vi "Optoelectronic Loop.vi"(8 "error in":errorcluster, 10 "Message Queues out":T14, 11 "Notifiers":T1) -> (0 "error out":errorcluster)   [LabVIEW 2014]
uses:
  support/Message Queue/All Message Queues.ctl
  support/Message Queue/Message Cluster.ctl
  support/Notifiers/Notifiers.ctl
  support/Message Handler Loop Notifiers.ctl
  Hardware Control/Parameter Analyzer/Parameter Analyzer Notifiers.ctl
  Hardware Control/Switching Matrix/Switching Matrix Notifiers.ctl
  Hardware Control/Stress Control/StressControl Notifiers.ctl
  Hardware Control/Spectrometer/Spectrometer Notifiers.ctl
  Hardware Control/Switches and Mirrors/SwitchesMirrors Notifiers.ctl
  Hardware Control/Camera/Camera Notifiers.ctl
  Hardware Control/XYZ Stage/XYZ Notifications.ctl
  Hardware Control/Autofocus/Autofocus Notifiers.ctl
  Measurements/Optoelectronic Measurement/Optoelectronic Notifiers.ctl
  Measurements/Save Data/SaveData Notifiers.ctl
  Measurements/Instrument Sequence/Instrument Sequence Notifiers.ctl
  Measurements/Optoelectronic Measurement/Optoelectronic Funtions.ctl
  support/Message Queue/Message Queue.lvlib
panel:
  # "LICENSED MATERIALS – PROPERTY OF IBM\nCopyright IBM Corp. 2016,\nALL RIGHTS RESERVED"
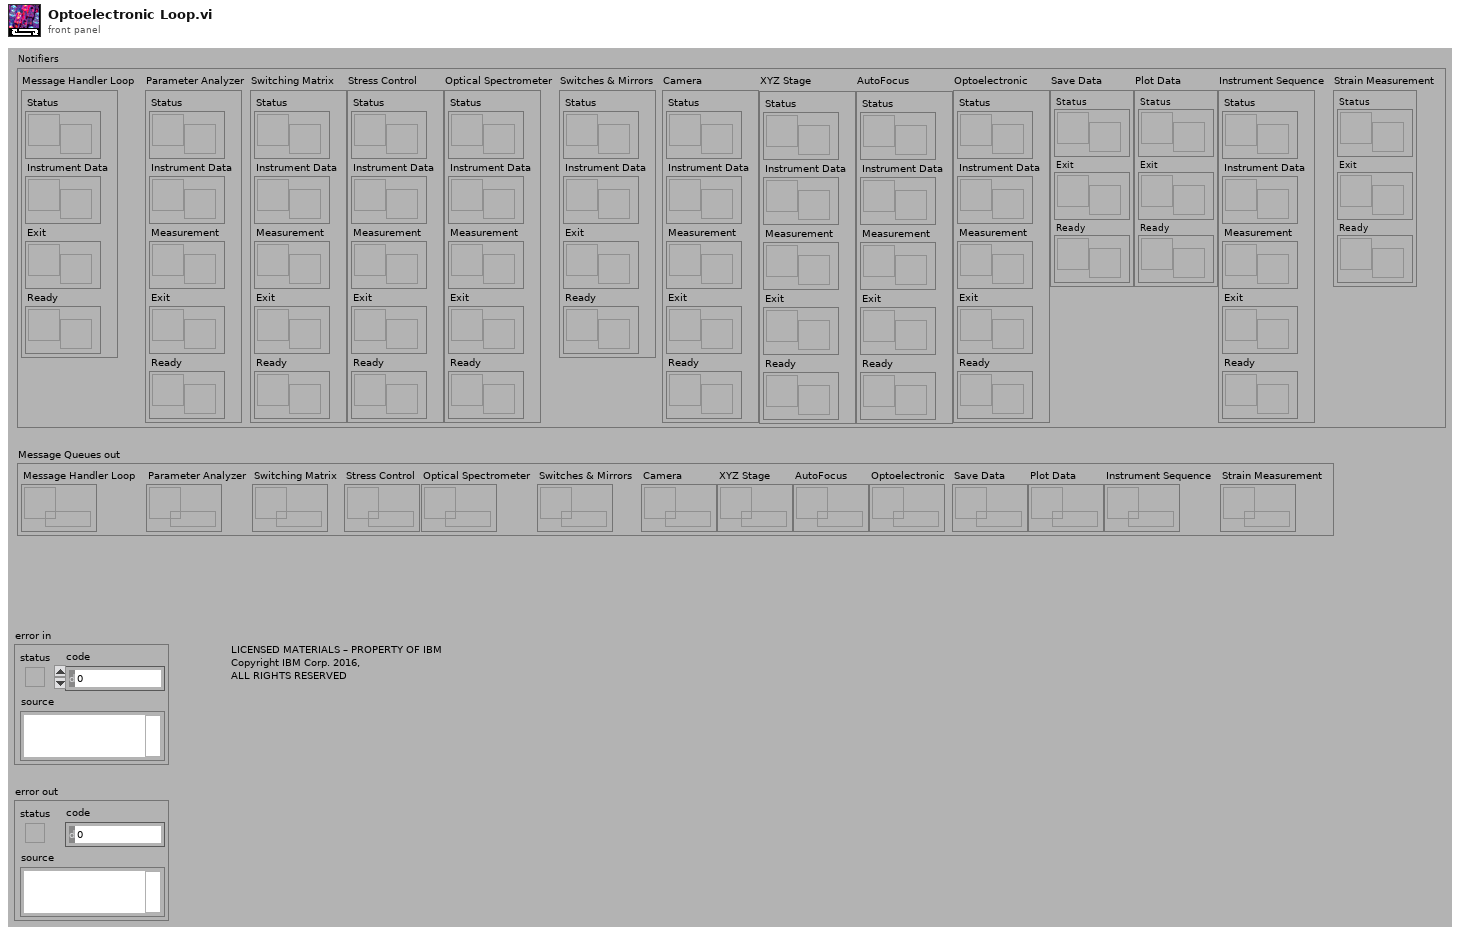
[diagram p1: front panel]
types:
  T1 = typedef "Notifiers.ctl" = cluster{"Message Handler Loop":T2, "Parameter Analyzer":T3, "Switching Matrix":T4, "Stress Control":T5, "Optical Spectrometer":T6, "Switches & Mirrors":T7, "Camera":T8, "XYZ Stage":T9, "AutoFocus":T10, "Optoelectronic":T11, "Save Data":T12, "Plot Data":T12, "Instrument Sequence":T13, "Strain Measurement":cluster{"Status":refnum<notifier>, "Exit":refnum<notifier>, "Ready":refnum<notifier>}}
  T2 = typedef "Message Handler Loop Notifiers.ctl" = cluster{"Status":refnum<notifier>, "Instrument Data":refnum<notifier>, "Exit":refnum<notifier>, "Ready":refnum<notifier>}
  T3 = typedef "Parameter Analyzer Notifiers.ctl" = cluster{"Status":refnum<notifier>, "Instrument Data":refnum<notifier>, "Measurement":refnum<notifier>, "Exit":refnum<notifier>, "Ready":refnum<notifier>}
  T4 = typedef "Switching Matrix Notifiers.ctl" = cluster{"Status":refnum<notifier>, "Instrument Data":refnum<notifier>, "Measurement":refnum<notifier>, "Exit":refnum<notifier>, "Ready":refnum<notifier>}
  T5 = typedef "StressControl Notifiers.ctl" = cluster{"Status":refnum<notifier>, "Instrument Data":refnum<notifier>, "Measurement":refnum<notifier>, "Exit":refnum<notifier>, "Ready":refnum<notifier>}
  T6 = typedef "Spectrometer Notifiers.ctl" = cluster{"Status":refnum<notifier>, "Instrument Data":refnum<notifier>, "Measurement":refnum<notifier>, "Exit":refnum<notifier>, "Ready":refnum<notifier>}
  T7 = typedef "SwitchesMirrors Notifiers.ctl" = cluster{"Status":refnum<notifier>, "Instrument Data":refnum<notifier>, "Exit":refnum<notifier>, "Ready":refnum<notifier>}
  T8 = typedef "Camera Notifiers.ctl" = cluster{"Status":refnum<notifier>, "Instrument Data":refnum<notifier>, "Measurement":refnum<notifier>, "Exit":refnum<notifier>, "Ready":refnum<notifier>}
  T9 = typedef "XYZ Notifications.ctl" = cluster{"Status":refnum<notifier>, "Instrument Data":refnum<notifier>, "Measurement":refnum<notifier>, "Exit":refnum<notifier>, "Ready":refnum<notifier>}
  T10 = typedef "Autofocus Notifiers.ctl" = cluster{"Status":refnum<notifier>, "Instrument Data":refnum<notifier>, "Measurement":refnum<notifier>, "Exit":refnum<notifier>, "Ready":refnum<notifier>}
  T11 = typedef "Optoelectronic Notifiers.ctl" = cluster{"Status":refnum<notifier>, "Instrument Data":refnum<notifier>, "Measurement":refnum<notifier>, "Exit":refnum<notifier>, "Ready":refnum<notifier>}
  T12 = typedef "SaveData Notifiers.ctl" = cluster{"Status":refnum<notifier>, "Exit":refnum<notifier>, "Ready":refnum<notifier>}
  T13 = typedef "Instrument Sequence Notifiers.ctl" = cluster{"Status":refnum<notifier>, "Instrument Data":refnum<notifier>, "Measurement":refnum<notifier>, "Exit":refnum<notifier>, "Ready":refnum<notifier>}
  T14 = typedef "Message Queue.lvlib/All Message Queues.ctl" = cluster{"Message Handler Loop":refnum<queue>, "Parameter Analyzer":refnum<queue>, "Switching Matrix":refnum<queue>, "Stress Control":refnum<queue>, "Optical Spectrometer":refnum<queue>, "Switches & Mirrors":refnum<queue>, "Camera":refnum<queue>, "XYZ Stage":refnum<queue>, "AutoFocus":refnum<queue>, "Optoelectronic":refnum<queue>, "Save Data":refnum<queue>, "Plot Data":refnum<queue>, "Instrument Sequence":refnum<queue>, "Strain Measurement":refnum<queue>}
  T15 = typedef "Optoelectronic Data.ctl" = cluster{"Refnums":T16, "Initialize":T19}
  T16 = typedef "Optoelectronic Refnums.ctl" = cluster{"Instrument Status":refnum<vi>, "Optical Spectrum Plot":T17, "Electrical Data Plot":T18}
  T17 = typedef "Optical Spectrum Plot Refnum.ctl" = cluster{"Plot List":refnum<vi>, "Optical Spectrum vs Energy":refnum<vi>, "Optical Spectrum vs Wavelength":refnum<vi>, "Optical Spectrum vs Raman Shift":refnum<vi>, "Detector Temperature":refnum<vi>}
  T18 = typedef "Electrical Data Plot Refnums.ctl" = cluster{"Plot List":refnum<vi>, "Voltage Plot":refnum<vi>, "Current Plot":refnum<vi>, "IV Characteristic":refnum<vi>, "dI/dV-V Characteristic":refnum<vi>}
  T19 = typedef "Optoelectronic Initialize.ctl" = cluster{"Update Refnums":bool}
  T20 = typedef "Optoelectronic Funtions.ctl" = enum16{"Get Instruments Status", "Measure", "Set Parameter Analyzer", "Set Spectrometer", "Set Acquisition", "Update Refnums"}
  T21 = typedef "SaveData Workspace Info.ctl" = cluster{"Device Name":string, "Device Info":string, "Path":path}
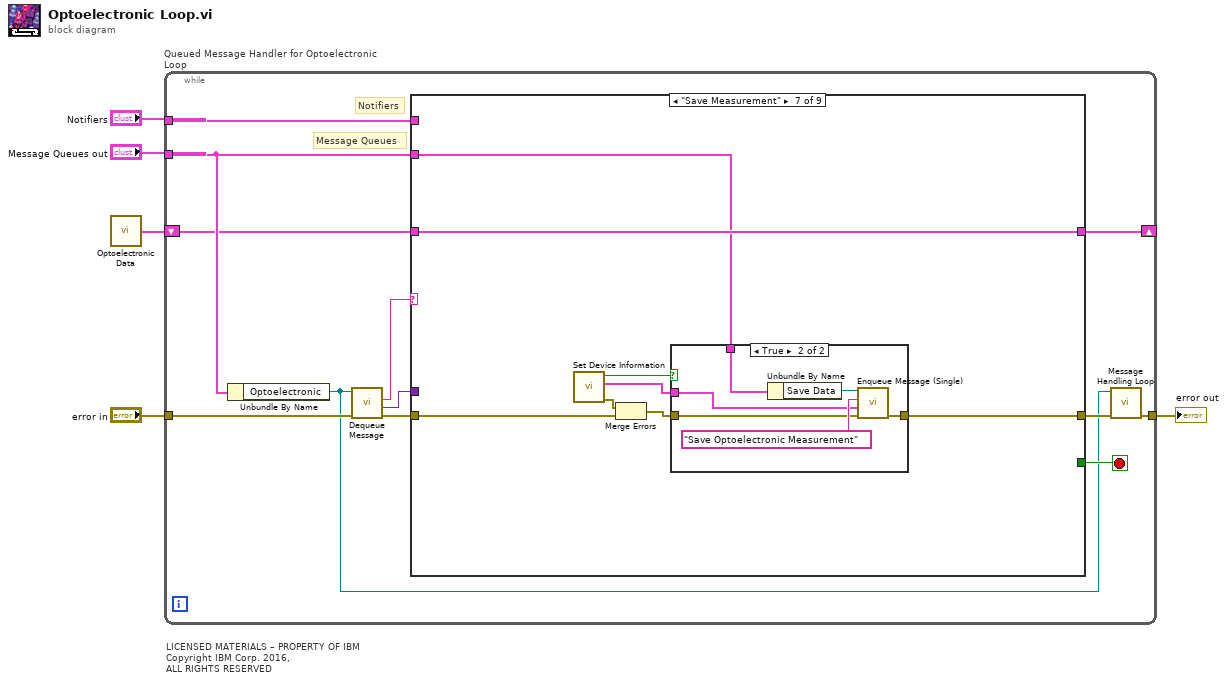
[diagram p0: block diagram]
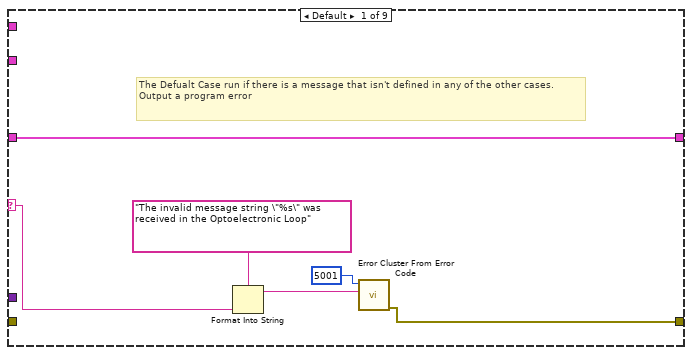
[diagram p2: hidden frame]
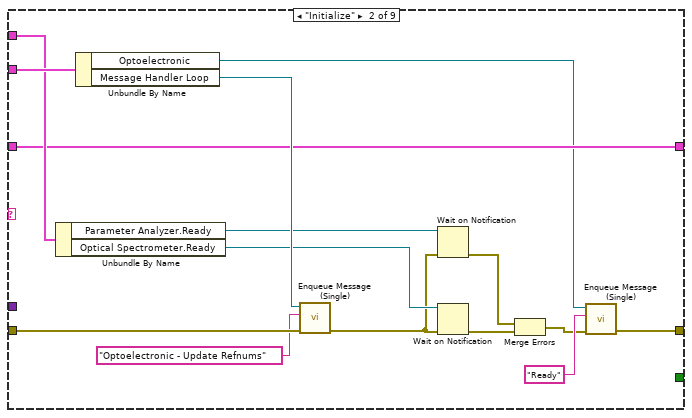
[diagram p3: hidden frame]
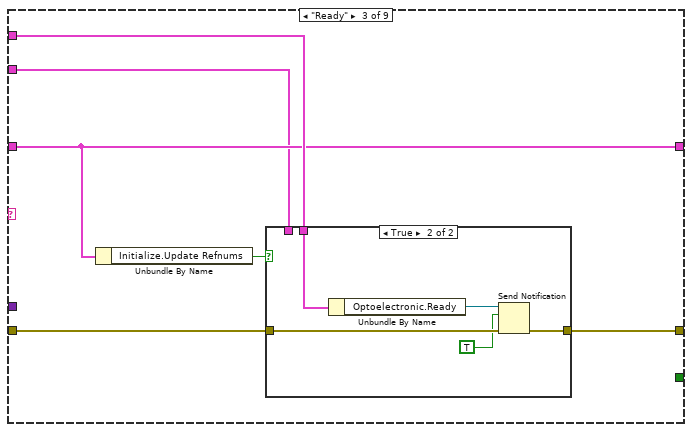
[diagram p4: hidden frame]
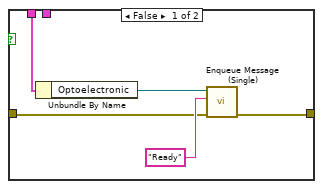
[diagram p5: hidden frame]
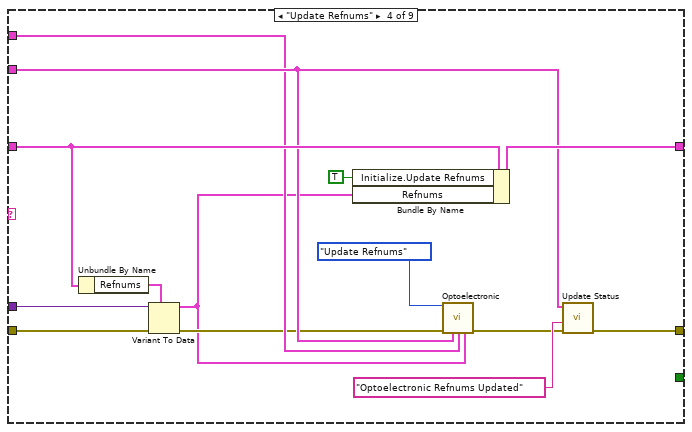
[diagram p6: hidden frame]
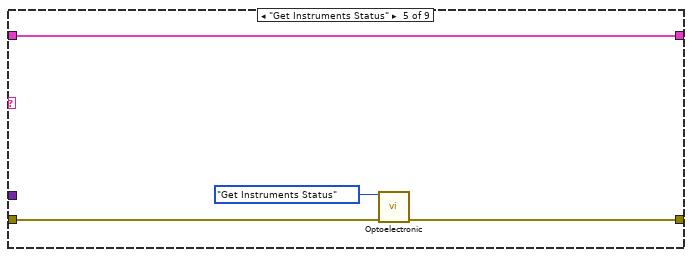
[diagram p7: hidden frame]
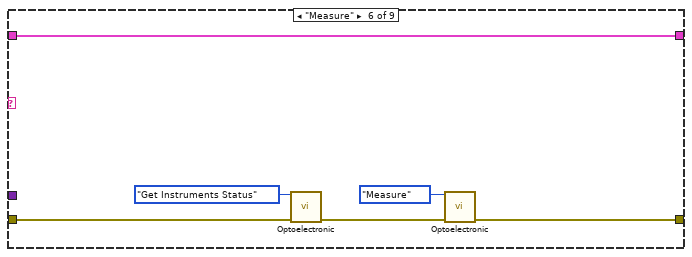
[diagram p8: hidden frame]
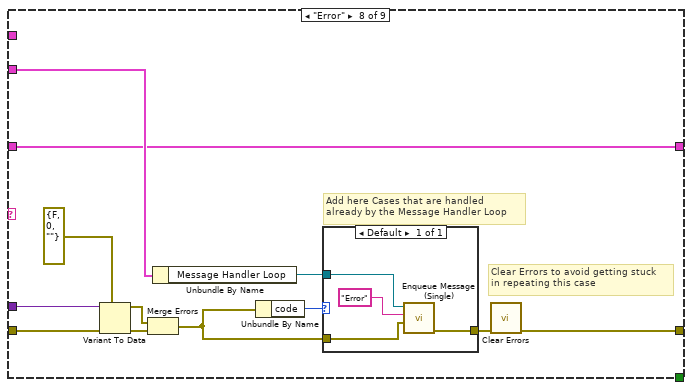
[diagram p10: hidden frame]
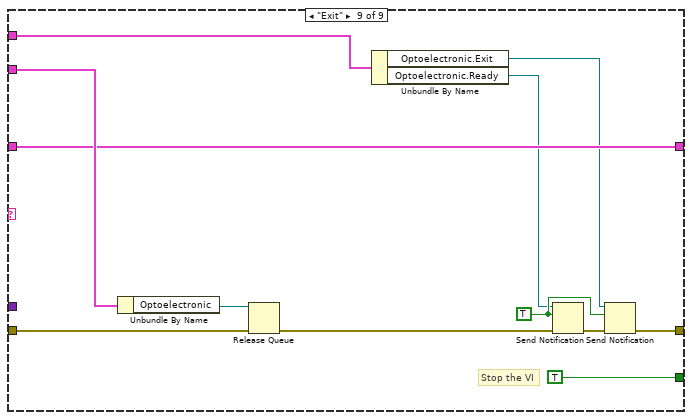
[diagram p11: hidden frame]
diagram:
  # "LICENSED MATERIALS – PROPERTY OF IBM\nCopyright IBM Corp. 2016,\nALL RIGHTS RESERVED"
  n1 = call "Optoelectronic Data.vi"() -> ("Optoelectronic Data"=w3:T15)
  n2 = while "Queued Message Handler for Optoelectronic Loop" {
    tunnel: "error in" -> [w17]
    tunnel: [w9] -> w1
    tunnel: "Message Queues out" -> [w13]
    tunnel: "Notifiers" -> [w12]
    shift-right: [w6] -> _
    shift-left: w3 -> [w7]
    stop <- w11 stop-if-true
    # "Notifiers"
    # "Message Queues"
    n3 = Unbundle By Name(w13) -> ("Optoelectronic"=w8:refnum<queue>)
    n4 = call "Dequeue Message.vi"("error in (no error)"=w17, "Message Queue"=w8) -> ("error out"=w16:errorcluster, "Message Data"=w14:variant, "Message"=w15:string)  [unwired: 7 out]
    n5 = case shown="\"Save Measurement\"" w15 {
      selector: w15 -> [w20 _ _ _ _ _ _ _ _]
      tunnel: w16 -> [_ w36 w42 w58 w70 w75 w81 w102 w117]
      tunnel: [w19 w27 w44 w68 w69 w77 w79 w97 w110] -> w10
      tunnel: w14 -> [_ _ _ w59 _ _ _ w95 _]
      tunnel: w13 -> [_ w38 w39 w62 _ _ w80 w103 w120]
      tunnel: w12 -> [_ w37 w43 w61 _ _ _ _ w112]
      tunnel: [_ _ _ _ _ _ _ _ TRUE ("Priority Message? (F)")] -> w11
      tunnel: w7 -> [w18 w32 w41 w66 w72 w78 w86 w94 w118]
      tunnel: [w18 w32 w41 w67 w72 w78 w86 w94 w118] -> w6
      frame Default {
        # "The Defualt Case run if there is a message that isn't defined in any of the other cases.\nOutput a program error"
        n6 = Format Into String(format string="The invalid message string \"%s\" was  received in the Optoelectronic Loop", w20) -> (resulting string=w22:string)  [unwired: 2 in, 1 out]
        n7 = call <vilib>:"Error Cluster From Error Code.vi"("error message (\"\")"=w22, "error code (0)"=5001) -> ("error out"=w19:errorcluster)  [unwired: 2 in, 5 out]
      }
      frame "Initialize" {
        n8 = Unbundle By Name(w37) -> ("Parameter Analyzer.Ready"=w33:refnum<notifier>, "Optical Spectrometer.Ready"=w31:refnum<notifier>)
        n9 = Unbundle By Name(w38) -> ("Optoelectronic"=w29:refnum<queue>, "Message Handler Loop"=w34:refnum<queue>)
        n10 = call "Enqueue Message (Single).vi"("error in (no error)"=w36, "Message"="Optoelectronic - Update Refnums", "Message Queue"=w34) -> ("error out"=w30:errorcluster)  [unwired: 1 in, 7 out]
        n11 = Wait on Notification(notifier=w33, error in (no error)=w30) -> (error out=w26:errorcluster)  [unwired: 5 out]
        n12 = Wait on Notification(notifier=w31, error in (no error)=w30) -> (error out=w25:errorcluster)  [unwired: 5 out]
        n13 = Merge Errors(w26, w25) -> (w24:errorcluster)
        n14 = call "Enqueue Message (Single).vi"("error in (no error)"=w24, "Message"="Ready", "Message Queue"=w29) -> ("error out"=w27:errorcluster)  [unwired: 1 in, 7 out]
      }
      frame "Ready" {
        n15 = Unbundle By Name(w41) -> ("Initialize.Update Refnums"=w40:bool)
        n16 = case shown="True" w40 {
          tunnel: [w45 w54] -> w44
          tunnel: w43 -> [_ w52]
          tunnel: w42 -> [w46 w51]
          tunnel: w39 -> [w48 _]
          frame False {
            n17 = Unbundle By Name(w48) -> ("Optoelectronic"=w47:refnum<queue>)
            n18 = call "Enqueue Message (Single).vi"("error in (no error)"=w46, "Message"="Ready", "Message Queue"=w47) -> ("error out"=w45:errorcluster)  [unwired: 1 in, 7 out]
          }
          frame True {
            n19 = Unbundle By Name(w52) -> ("Optoelectronic.Ready"=w53:refnum<notifier>)
            n20 = Send Notification(notification=TRUE, notifier=w53, error in (no error)=w51) -> (error out=w54:errorcluster)  [unwired: 1 out]
          }
        }
      }
      frame "Update Refnums" {
        n21 = Unbundle By Name(w66) -> ("Refnums"=w56:T16)
        n22 = Variant To Data(error in=w58, type=w56, Variant=w59) -> (data=w55:T16, error out=w57:errorcluster)
        n23 = Bundle By Name(cluster=w66, "Initialize.Update Refnums"=TRUE, "Refnums"=w55) -> (w67:T15)
        n24 = call "Optoelectronic.vi"("Function"=Optoelectronic_Funtions."Update Refnums", "error in (no error)"=w57, "Message Queues"=w62, "Notifiers"=w61, "Refnums"=w55) -> ("error out"=w63:errorcluster)  [unwired: 10 in]
        n25 = call "Update Status.vi"("error in"=w63, "String"="Optoelectronic Refnums Updated", "Message Queues out"=w62) -> ("error out"=w68:errorcluster)  [unwired: 8 out]
      }
      frame "Get Instruments Status" {
        n26 = call "Optoelectronic.vi"("Function"=Optoelectronic_Funtions."Get Instruments Status", "error in (no error)"=w70) -> ("error out"=w69:errorcluster)  [unwired: 13 in]
      }
      frame "Measure" {
        n27 = call "Optoelectronic.vi"("Function"=Optoelectronic_Funtions."Get Instruments Status", "error in (no error)"=w75) -> ("error out"=w76:errorcluster)  [unwired: 13 in]
        n28 = call "Optoelectronic.vi"("Function"=Optoelectronic_Funtions."Measure", "error in (no error)"=w76) -> ("error out"=w77:errorcluster)  [unwired: 13 in]
      }
      frame "Save Measurement" {
        n29 = call "Set Device Information.vi"() -> ("error out"=w83:errorcluster, "Workspace Info"=w82:T21, "OK?"=w85:bool)  [unwired: 1 in, 8 out]
        n30 = Merge Errors(w83, w81) -> (w84:errorcluster)
        n31 = case shown="True" w85 {
          tunnel: w80 -> [_ w91]
          tunnel: w84 -> [w87 w90]
          tunnel: [w87 w89] -> w79
          tunnel: w82 -> [_ w88]
          frame False {
          }
          frame True {
            n32 = Unbundle By Name(w91) -> ("Save Data"=w92:refnum<queue>)
            n33 = call "Enqueue Message (Single).vi"("error in (no error)"=w90, "Message Data"=w88, "Message"="Save Optoelectronic Measurement", "Message Queue"=w92) -> ("error out"=w89:errorcluster)  [unwired: 7 out]
          }
        }
      }
      frame "Error" {
        # "Clear Errors to avoid getting stuck \nin repeating this case"
        # "Add here Cases that are handled \nalready by the Message Handler Loop"
        n34 = Variant To Data(error in=w102, type=errorcluster {"status"=FALSE, "code"=0, "source"=""} ("error out"), Variant=w95) -> (data=w101:errorcluster, error out=w100:errorcluster)
        n35 = Merge Errors(w101, w100) -> (w99:errorcluster)
        n36 = Unbundle By Name(w103) -> ("Message Handler Loop"=w105:refnum<queue>)
        n37 = Unbundle By Name(w99) -> ("code"=w96:i32)
        n38 = case shown="Default" w96 {
          tunnel: w105 -> [w109]
          tunnel: w99 -> [w107]
          tunnel: [w106] -> w98
          frame Default {
            n39 = call "Enqueue Message (Single).vi"("Message Data"=w107, "Message"="Error", "Message Queue"=w109) -> ("error out"=w106:errorcluster)  [unwired: 1 in, 7 out]
          }
        }
        n40 = call <vilib>:"Clear Errors.vi"("error in (no error)"=w98) -> ("error out"=w97:errorcluster)  [unwired: 1 in, 5 out]
      }
      frame "Exit" {
        w115 = TRUE ("Priority Message? (F)")
        # "Stop the VI"
        n41 = Unbundle By Name(w120) -> ("Optoelectronic"=w121:refnum<queue>)
        n42 = Release Queue(queue=w121, error in (no error)=w117) -> (error out=w111:errorcluster)  [unwired: 3 out]
        n43 = Unbundle By Name(w112) -> ("Optoelectronic.Exit"=w116:refnum<notifier>, "Optoelectronic.Ready"=w113:refnum<notifier>)
        n44 = Send Notification(notification=w115, notifier=w113, error in (no error)=w111) -> (error out=w114:errorcluster)  [unwired: 1 out]
        n45 = Send Notification(notification=w115, notifier=w116, error in (no error)=w114) -> (error out=w110:errorcluster)  [unwired: 1 out]
      }
    }
    n46 = call "Message Handling Loop.vi"("error in (no error)"=w10, "Message Queue"=w8) -> ("dup error in"=w9:errorcluster)  [unwired: 9 out]
  }
  "error out" <- w1
